vi "shiftregisters_counters.vi"() -> ()   [LabVIEW 2016]
panel:
  out "Array":dbl[](array[numeric])
  out "Array 2":dbl[][](array[numeric])
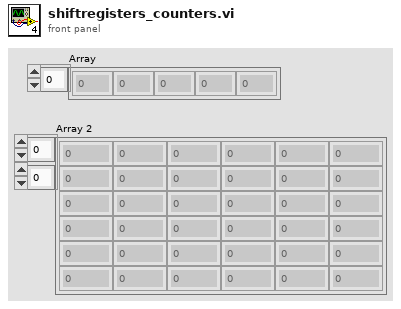
[diagram p1: front panel]
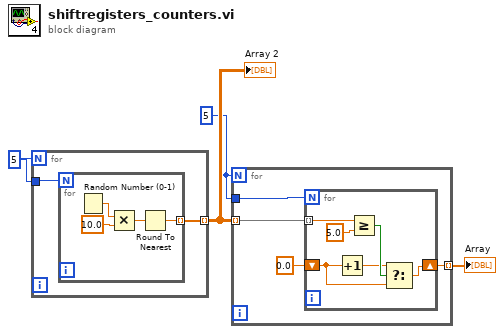
[diagram p0: block diagram]
diagram:
  w4 = 5
  w2 = 5
  n1 = for {
    N: w4 -> [_]
    tunnel: w4 -> [w6]
    tunnel: [w5] -> w3 mode=indexing
    n2 = for {
      N: w6 -> [_]
      tunnel: [w7] -> w5 mode=indexing
      n3 = Random Number (0-1)() -> (number: 0 to 1=w10:dbl)
      n4 = Multiply(x=w10, y=10.0) -> (x*y=w8:dbl)
      n5 = Round To Nearest(number=w8) -> (nearest integer value=w7:dbl)
    }
  }
  "Array 2" <- w3
  n6 = for {
    N: w2 -> [_]
    tunnel: w3 -> [w14] mode=indexing
    tunnel: w2 -> [w13]
    tunnel: [w11] -> w1 mode=indexing
    n7 = for {
      N: w13 -> [_]
      tunnel: w14 -> [w20] mode=indexing
      shift-right: [w16] -> w11
      shift-left: 0.0 -> [w15]
      n8 = Increment(x=w15) -> (x+1=w17:dbl)
      n9 = Greater Or Equal?(x=w20, y=5.0) -> (x >= y?=w18:bool)
      n10 = Select(t=w17, s=w18, f=w15) -> (s? t:f=w16:dbl)
    }
  }
  "Array" <- w1
